vi "ClassAttributes_GetClassAttributes_4x4x4.vi"(8 "error in (no error)":errorcluster, 11 "reference in":refnum<class>) -> (0 "error out":errorcluster, 1 "Class attribute Reference":refnum<data-value>, 2 "Class attribute":T1, 3 "reference out":refnum<class>)   [LabVIEW 2010]
doc: "Returns the class attributes of this class or a sub class. If reference is wired, the class attributes of the class (or sub class) will be returned else the class attributes will default to this class.\n\nIf the data is currently locked for modification, 'Attributes locked?' will return TRUE. If reference is wired, the class attributes of this class (or sub class) will be returned else the class attributes of this class."
uses:
  ClassAttributes_ClassAttributes.ctl
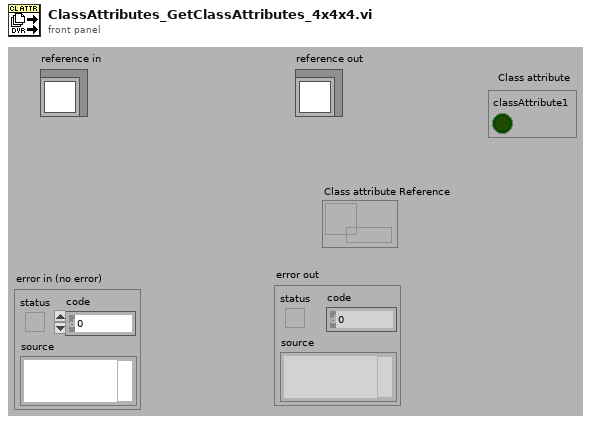
[diagram p1: front panel]
types:
  T1 = typedef "ClassAttributes_ClassAttributes.ctl" = cluster{"classAttribute1":bool}
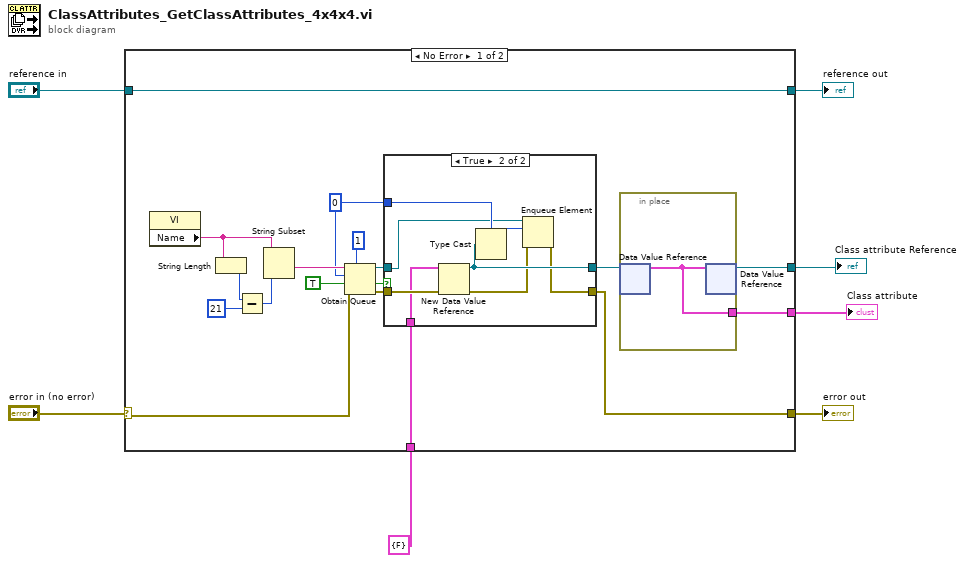
[diagram p0: block diagram]
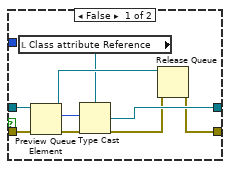
[diagram p2: hidden frame]
diagram:
  n1 = case shown="No Error" "error in (no error)" {
    selector: "error in (no error)" -> [w14 w43]
    tunnel: [w25 w44] -> w7
    tunnel: [w13 w43] -> w6
    tunnel: "reference in" -> [w25 w44]
    tunnel: T1 {"classAttribute1"=FALSE} ("Class attributes") -> [w16 _]
    tunnel: [w11 _] -> w2
    tunnel: [w10 _] -> w1
    frame No Error {
      w9 = u32 0 ("max queue size (-1, unlimited)")
      n2 = property class="VI"() -> ("Name"=w8:string)  [unwired: 2 in, 2 out]
      n3 = String Length(string=w8) -> (length=w24:i32)
      n4 = Subtract(x=w24, y=21) -> (x-y=w22:i32)
      n5 = String Subset(string=w8, length (rest)=w22) -> (substring=w21:string)  [unwired: 1 in]
      n6 = Obtain Queue(max queue size (-1, unlimited)=1, name (unnamed)=w21, element data type=w9, create if not found? (T)=TRUE, error in (no error)=w14) -> (queue out=w15:refnum<queue>, created new?=w18:bool, error out=w17:errorcluster)
      n7 = case shown="True" w18 {
        tunnel: w17 -> [w34 w42]
        tunnel: w16 -> [_ w41]
        tunnel: w15 -> [w33 w38]
        tunnel: [w31 w40] -> w12
        tunnel: [w28 w35] -> w13
        tunnel: w9 -> [_ w39]
        frame False {
          n8 = local read "Class attribute Reference"() -> (w27:refnum<data-value>)
          n9 = Preview Queue Element(queue=w33, error in (no error)=w34) -> (queue out=w30:refnum<queue>, element=w32:u32, error out=w29:errorcluster)  [unwired: 1 in, 1 out]
          n10 = Type Cast(type=w27, x=w32) -> (*(type *) &x=w31:refnum<data-value>)
          n11 = Release Queue(queue=w30, error in (no error)=w29) -> (error out=w28:errorcluster)  [unwired: 1 in, 2 out]
        }
        frame True {
          n12 = New Data Value Reference(data value=w41, error in=w42) -> (data value reference=w40:refnum<data-value>, error out=w36:errorcluster)
          n13 = Type Cast(type=w39, x=w40) -> (*(type *) &x=w37:u32)
          n14 = Enqueue Element(queue=w38, element=w37, error in (no error)=w36) -> (error out=w35:errorcluster)  [unwired: 1 in, 2 out]
        }
      }
      n15 = in-place {
        in-place-border: [w26] -> w10
        n16 = in-place-dvr #1(w12) -> (w26:T1)  [unwired: 1 out]
        n17 = in-place-dvr #1(w26) -> (w11:refnum<data-value>)  [unwired: 1 out]
      }
    }
    frame Error {
    }
  }
  "error out" <- w6
  "reference out" <- w7
  "Class attribute" <- w1
  "Class attribute Reference" <- w2
